vi "g-secrets.vi"   [LabVIEW 2025]
doc: "This VI is a CLI interface that wraps the core VIs of the G-Secrets project to allow secret scanning of LabVIEW Code."
uses:
  Type Definitions/CLI States--enum.ctl
  Type Definitions/CLI Data--cluster.ctl
  <vilib>/Wiresmith Technology/G CLI/CLI Class/CLI.lvclass
  <vilib>/Utility/error.llb/DialogType.ctl
  <userlib>/_OpenG.lib/file/file.llb/File Exists - Scalar__ogtk.vi
  <userlib>/_OpenG.lib/file/file.llb/openg_file.lvlib
types:
  T1 = typedef "CLI Data--cluster.ctl" = cluster{"File":path, "Help":bool, "Export Only":bool, "Quiet":bool, "Include Secrets":bool, "String File":path, "Log File":path, "Report File":path, "CLI Reference":refnum<class "CLI.lvclass">, "CLI Custom Parameters":string[], "Exit Code":i32, "Secrets Config":path}
  T2 = typedef "CLI States--enum.ctl" = enum16{"Initialize", "Help Message", "Export Strings", "Find Secrets", "Error", "Exit"}
  T3 = enum16{"open", "replace", "create", "open or create", "replace or create", "replace or create with confirmation"}
  T4 = typedef "Option Parser.lvlib/Option.lvclass/Option Configuration.ctl" = cluster{"Option Type":T5, "Option Labels":string[], "Key":string, "Description":string, "Required":bool, "Default Value":string}
  T5 = typedef "Option Parser.lvlib/Option.lvclass/Argument Type.ctl" = enum16{"flag", "value"}
  T6 = typedef "Leak--cluster.ctl" = cluster{"Secret":T7, "Value":string}
  T7 = typedef "Secret--cluster.ctl" = cluster{"Name":string, "Regex":string}
  T8 = typedef "DialogType.ctl" = u16
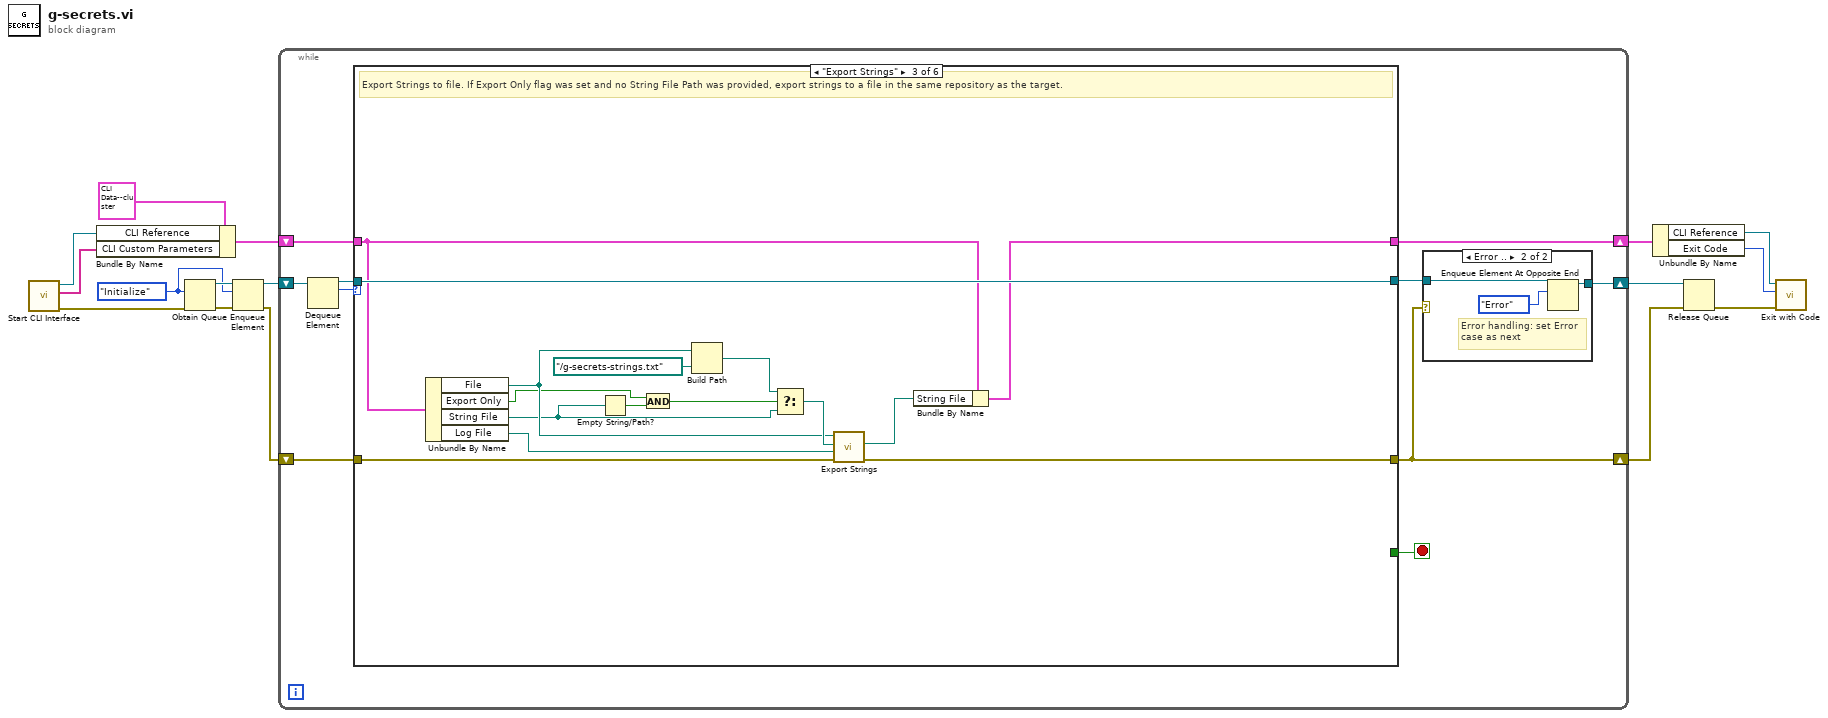
[diagram p0: block diagram]
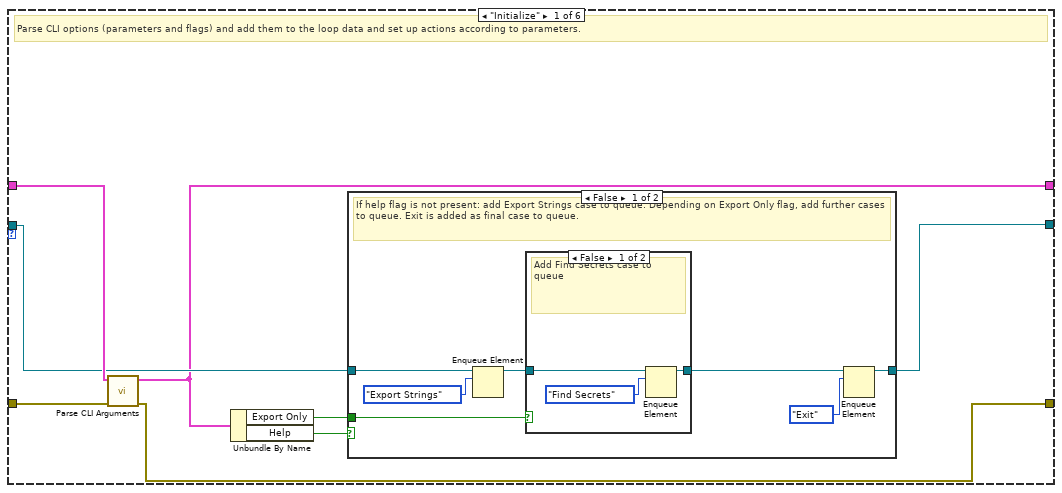
[diagram p3: hidden frame]
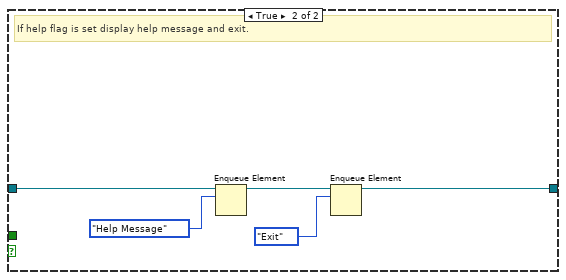
[diagram p5: hidden frame]
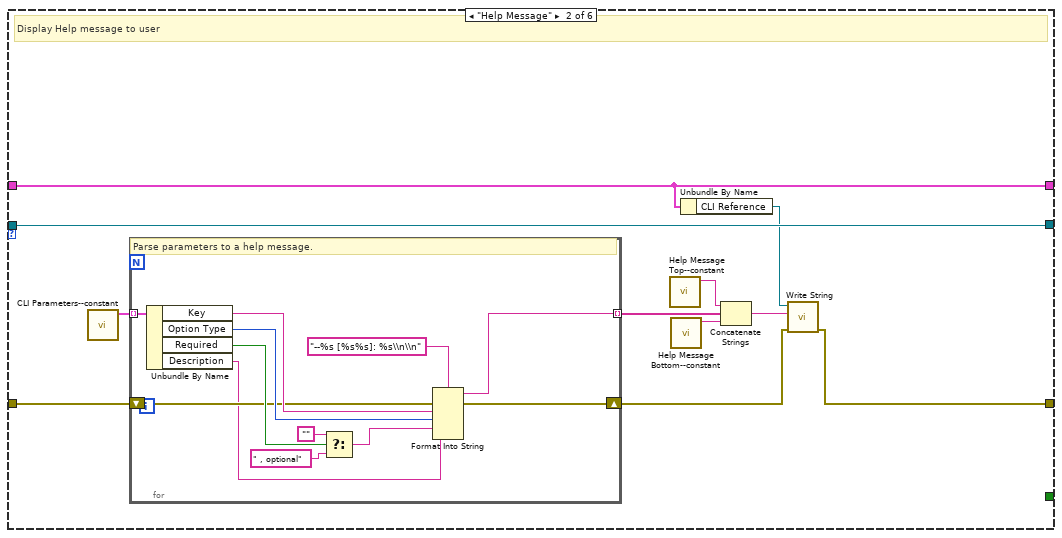
[diagram p6: hidden frame]
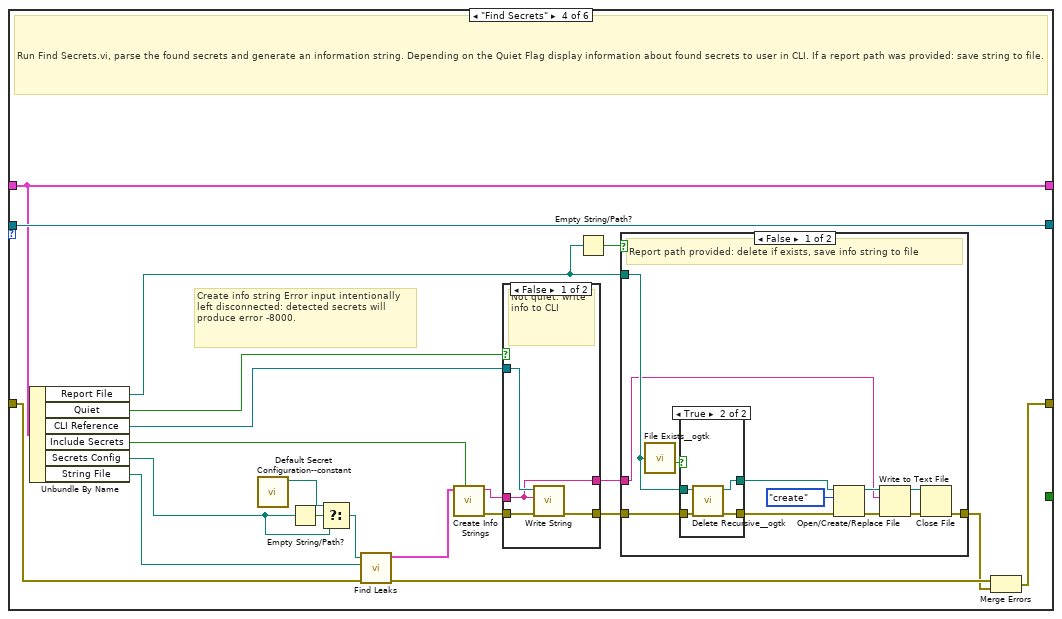
[diagram p7: hidden frame]
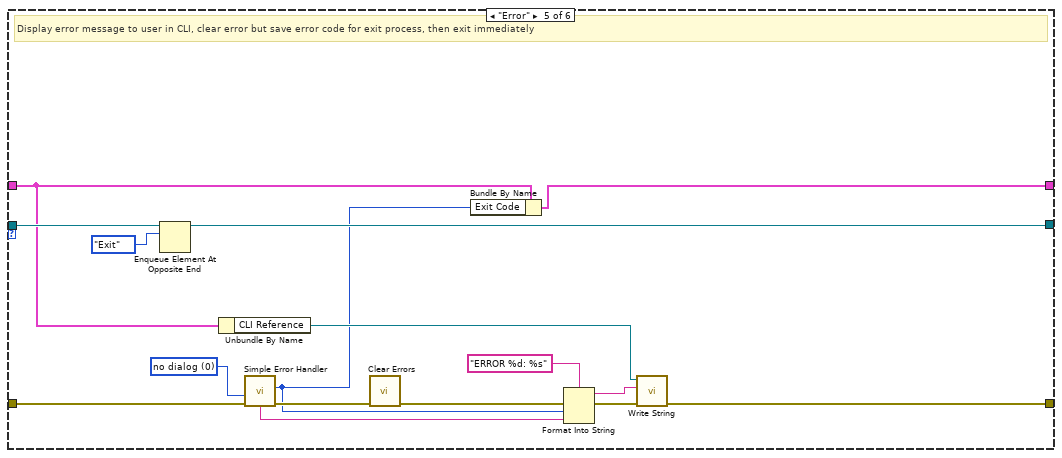
[diagram p11: hidden frame]
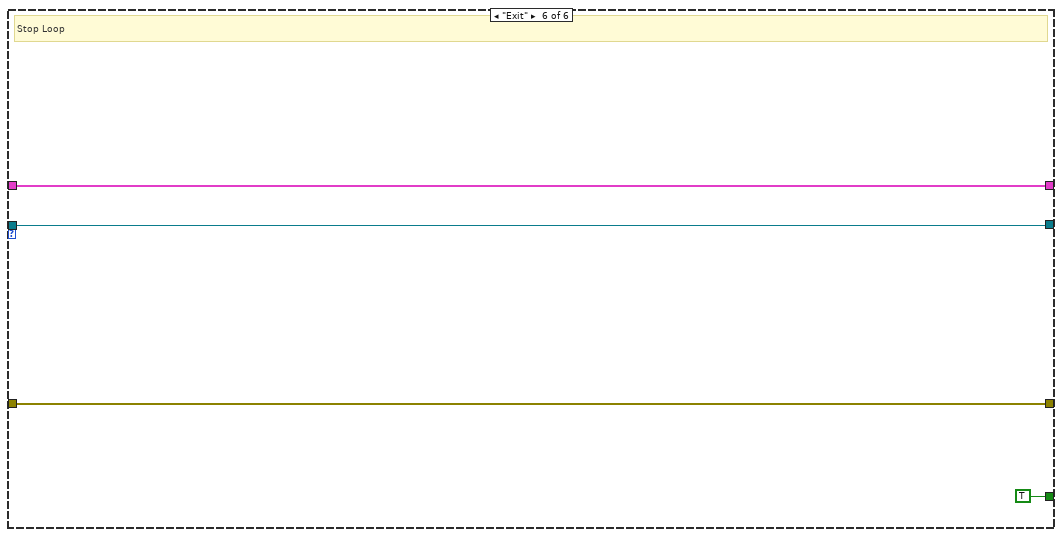
[diagram p12: hidden frame]
diagram:
  w13 = CLI_States--enum."Initialize"
  n1 = call <vilib>:"Start CLI Interface.vi"() -> ("error out"=w12:errorcluster, "Custom Parameters"=w9:string[], "CLI out"=w10:refnum<class "CLI.lvclass">)  [unwired: 8 in, 1 out]
  n2 = Bundle By Name(cluster=T1 {"File"=path "", "Help"=FALSE, "Export Only"=FALSE, "Quiet"=FALSE, "Include Secrets"=FALSE, "String File"=path "", "Log File"=path "", "Report File"=path "", "CLI Reference"=refnum, "CLI Custom Parameters"=[], "Exit Code"=0, "Secrets Config"=path ""} ("CLI Data"), "CLI Reference"=w10, "CLI Custom Parameters"=w9) -> (w8:T1)
  n3 = Obtain Queue(element data type=w13, error in (no error)=w12) -> (queue out=w16:refnum<queue>, error out=w14:errorcluster)  [unwired: 3 in, 1 out]
  n4 = Enqueue Element(queue=w16, element=w13, error in (no error)=w14) -> (queue out=w15:refnum<queue>, error out=w7:errorcluster)  [unwired: 1 in, 1 out]
  n5 = while {
    shift-right: [w19] -> w6
    shift-left: w15 -> [w25]
    shift-right: [w18] -> w5
    shift-left: w7 -> [w26]
    shift-right: [w21] -> w3
    shift-left: w8 -> [w22]
    stop <- w17 stop-if-true
    n6 = Dequeue Element(queue=w25) -> (queue out=w23:refnum<queue>, element=w24:T2)  [unwired: 2 in, 2 out]
    n7 = case shown="\"Export Strings\"" w24 {
      tunnel: w26 -> [w38 w61 w91 w113 w151 w156]
      tunnel: w23 -> [w35 w60 w90 w104 w154 w157]
      tunnel: w22 -> [w37 w59 w88 w95 w146 w158]
      tunnel: [w34 w59 w89 w95 w148 w158] -> w21
      tunnel: [w31 w55 w87 w106 w147 w156] -> w18
      tunnel: [w32 w60 w90 w104 w152 w157] -> w20
      tunnel: [_ _ _ _ _ TRUE] -> w17
      frame "Initialize" {
        # "Parse CLI options (parameters and flags) and add them to the loop data and set up actions according to parameters."
        n8 = call "Parse CLI Arguments.vi"("error in"=w38, "CLI Data in"=w37) -> ("error out"=w31:errorcluster, "CLI Data out"=w34:T1)  [unwired: 4 in]
        n9 = Unbundle By Name(w34) -> ("Export Only"=w33:bool, "Help"=w36:bool)
        n10 = case shown="False" w36 {
          tunnel: w35 -> [w45 w54]
          tunnel: [w41 w50] -> w32
          tunnel: w33 -> [w39 _]
          frame False {
            # "If help flag is not present: add Export Strings case to queue. Depending on Export Only flag, add further cases to queue. Exit is added as final case to queue."
            n11 = Enqueue Element(queue=w45, element=CLI_States--enum."Export Strings") -> (queue out=w43:refnum<queue>)  [unwired: 2 in, 2 out]
            n12 = case shown="False" w39 {
              tunnel: w43 -> [w47 w49]
              tunnel: [w46 w49] -> w42
              frame False {
                # "Add Find Secrets case to queue"
                n13 = Enqueue Element(queue=w47, element=CLI_States--enum."Find Secrets") -> (queue out=w46:refnum<queue>)  [unwired: 2 in, 2 out]
              }
              frame True {
                # "Export only: no further actions"
              }
            }
            n14 = Enqueue Element(queue=w42, element=CLI_States--enum."Exit") -> (queue out=w41:refnum<queue>)  [unwired: 2 in, 2 out]
          }
          frame True {
            # "If help flag is set display help message and exit."
            n15 = Enqueue Element(queue=w54, element=CLI_States--enum."Help Message") -> (queue out=w51:refnum<queue>)  [unwired: 2 in, 2 out]
            n16 = Enqueue Element(queue=w51, element=CLI_States--enum."Exit") -> (queue out=w50:refnum<queue>)  [unwired: 2 in, 2 out]
          }
        }
      }
      frame "Help Message" {
        # "Display Help message to user"
        n17 = call "CLI Parameters--constant.vi"() -> ("CLI Parameters"=w65:T4[])  [unwired: 7 in]
        n18 = for {
          tunnel: w65 -> [w77] mode=indexing
          tunnel: [w66] -> w63 mode=indexing
          shift-right: [w68] -> w56
          shift-left: w61 -> [w69]
          # "Parse parameters to a help message."
          n19 = Unbundle By Name(w77) -> ("Key"=w75:string, "Option Type"=w74:T5, "Required"=w73:bool, "Description"=w67:string)
          n20 = Select(t="", s=w73, f=" , optional") -> (s? t:f=w70:string)
          n21 = Format Into String(format string="--%s [%s%s]: %s\\n\\n", error in=w69, w75, w74, w70, w67) -> (resulting string=w66:string, error out=w68:errorcluster)  [unwired: 1 in]
        }
        n22 = call "Help Message Top--constant.vi"() -> ("Help Message Top"=w64:string)  [unwired: 7 in]
        n23 = call "Help Message Bottom--constant.vi"() -> ("Help Message Bottom"=w62:string)  [unwired: 7 in]
        n24 = Unbundle By Name(w59) -> ("CLI Reference"=w58:refnum<class "CLI.lvclass">)
        n25 = Concatenate Strings(w64, w63, w62) -> (w57:string)
        n26 = call <vilib>:"Write String.vi"("error in (no error)"=w56, "Text to Write"=w57, "CLI in"=w58) -> ("error out"=w55:errorcluster)  [unwired: 7 in, 1 out]
      }
      frame "Export Strings" {
        # "Export Strings to file. If Export Only flag was set and no String File Path was provided, export strings to a file in the same repository as the target."
        n27 = Unbundle By Name(w88) -> ("File"=w83:path, "Export Only"=w79:bool, "String File"=w81:path, "Log File"=w92:path)
        n28 = Empty String/Path?(string/path=w81) -> (empty?=w80:bool)
        n29 = And(x=w79, y=w80) -> (x .and. y?=w78:bool)
        n30 = Build Path(base path=w83, name or relative path=path "../g-secrets-strings.txt") -> (appended path=w85:path)
        n31 = Select(t=w85, s=w78, f=w81) -> (s? t:f=w84:path)
        n32 = call "Export Strings.vi"("error in"=w91, "Log File"=w92, "String File"=w84, "Target"=w83) -> ("error out"=w87:errorcluster, "String File Out"=w82:path)  [unwired: 1 in, 1 out]
        n33 = Bundle By Name(cluster=w88, "String File"=w82) -> (w89:T1)
      }
      frame "Find Secrets" {
        # "Create info string Error input intentionally left disconnected: detected secrets will produce error -8000."
        # "Run Find Secrets.vi, parse the found secrets and generate an information string. Depending on the Quiet Flag display information about found secrets to user in CLI. If a report path was provided: save string to file."
        n34 = Unbundle By Name(w95) -> ("Report File"=w94:path, "Quiet"=w103:bool, "CLI Reference"=w105:refnum<class "CLI.lvclass">, "Include Secrets"=w112:bool, "Secrets Config"=w96:path, "String File"=w107:path)
        n35 = call "Default Secret Configuration--constant.vi"() -> ("Path"=w110:path)  [unwired: 7 in]
        n36 = Empty String/Path?(string/path=w96) -> (empty?=w111:bool)
        n37 = Select(t=w110, s=w111, f=w96) -> (s? t:f=w109:path)
        n38 = call "Find Leaks.vi"("error in"=w113, "String File"=w107, "Secrets Configuration"=w109) -> ("error out"=w108:errorcluster, "Leaks"=w93:T6[])  [unwired: 2 in, 1 out]
        n39 = call "Create Info Strings.vi"("Include Secrets"=w112, "Leaks"=w93) -> ("error out"=w100:errorcluster, "Info String"=w102:string)  [unwired: 6 in]
        n40 = case shown="False" w103 {
          tunnel: w105 -> [w136 _]
          tunnel: w102 -> [w133 w137]
          tunnel: w100 -> [w135 w138]
          tunnel: [w134 w138] -> w99
          tunnel: [w133 w137] -> w98
          frame False {
            # "Not quiet: write info to CLI"
            n41 = call <vilib>:"Write String.vi"("error in (no error)"=w135, "Text to Write"=w133, "CLI in"=w136) -> ("error out"=w134:errorcluster)  [unwired: 7 in, 1 out]
          }
          frame True {
            # "Quiet mode"
          }
        }
        n42 = Empty String/Path?(string/path=w94) -> (empty?=w101:bool)
        n43 = case shown="False" w101 {
          tunnel: w99 -> [w117 w132]
          tunnel: w98 -> [w115 _]
          tunnel: [w120 w132] -> w97
          tunnel: w94 -> [w118 _]
          frame False {
            # "Report path provided: delete if exists, save info string to file"
            n44 = call-poly <userlib>:"File Exists__ogtk.vi"("file path"=w118) -> ("exists"=w119:bool)  [unwired: 6 in, 1 out]
            n45 = case shown="True" w119 {
              tunnel: w118 -> [w126 w131]
              tunnel: w117 -> [w127 w130]
              tunnel: [w127 w129] -> w116
              tunnel: [w126 w128] -> w114
              frame False {
              }
              frame True {
                n46 = call <userlib>:"Delete Recursive__ogtk.vi"("error in (no error)"=w130, "Path"=w131) -> ("error out"=w129:errorcluster, "dup Path"=w128:path)  [unwired: 8 in]
              }
            }
            n47 = Open/Create/Replace File(file path (use dialog)=w114, error in=w116, operation (0:open)=T3."create") -> (refnum out=w123:refnum<file>, error out=w124:errorcluster)  [unwired: 3 in, 1 out]
            n48 = Write to Text File(file (use dialog)=w123, text=w115, error in=w124) -> (refnum out=w121:refnum<file>, error out=w122:errorcluster)  [unwired: 1 in, 1 out]
            n49 = Close File(refnum=w121, error in=w122) -> (error out=w120:errorcluster)  [unwired: 1 out]
          }
          frame True {
            # "No report path provided."
          }
        }
        n50 = Merge Errors(w108, w97) -> (w106:errorcluster)
      }
      frame "Error" {
        w150 = T8 0 items=["no dialog", "OK message", "continue or stop message", "OK message + warnings", "continue/stop + warnings"] ("type of dialog (OK msg:1)")
        # "Display error message to user in CLI, clear error but save error code for exit process, then exit immediately"
        n51 = Enqueue Element At Opposite End(queue=w154, element=CLI_States--enum."Exit") -> (queue out=w152:refnum<queue>)  [unwired: 2 in, 2 out]
        n52 = Unbundle By Name(w146) -> ("CLI Reference"=w145:refnum<class "CLI.lvclass">)
        n53 = call <vilib>:"Simple Error Handler.vi"("type of dialog (OK msg:1)"=w150, "error in (no error)"=w151) -> ("code out"=w141:i32, "error out"=w149:errorcluster, "message"=w140:string)  [unwired: 3 in, 2 out]
        n54 = call <vilib>:"Clear Errors.vi"("error in (no error)"=w149) -> ("error out"=w143:errorcluster)  [unwired: 5 in, 1 out]
        n55 = Bundle By Name(cluster=w146, "Exit Code"=w141) -> (w148:T1)
        n56 = Format Into String(format string="ERROR %d: %s", error in=w143, w141, w140) -> (resulting string=w139:string, error out=w142:errorcluster)  [unwired: 1 in]
        n57 = call <vilib>:"Write String.vi"("error in (no error)"=w142, "Text to Write"=w139, "CLI in"=w145) -> ("error out"=w147:errorcluster)  [unwired: 7 in, 1 out]
      }
      frame "Exit" {
        # "Stop Loop"
      }
    }
    n58 = case shown="Error .." w18 {
      tunnel: w20 -> [w27 w30]
      tunnel: [w27 w28] -> w19
      frame No Error {
      }
      frame Error {
        # "Error handling: set Error\ncase as next"
        n59 = Enqueue Element At Opposite End(queue=w30, element=CLI_States--enum."Error") -> (queue out=w28:refnum<queue>)  [unwired: 2 in, 2 out]
      }
    }
  }
  n60 = Unbundle By Name(w3) -> ("CLI Reference"=w1:refnum<class "CLI.lvclass">, "Exit Code"=w2:i32)
  n61 = Release Queue(queue=w6, error in (no error)=w5) -> (error out=w4:errorcluster)  [unwired: 1 in, 2 out]
  n62 = call <vilib>:"Exit with Code.vi"("error in (no error)"=w4, "Exit Code (0)"=w2, "CLI in"=w1) -> ()  [unwired: 8 in, 1 out]
